vi "IMAQ Multi-camera acquisition of images.vi"() -> ()   [LabVIEW 2018]
uses:
  LabViewDVPCamera/LabViewDVPCamera.lvlib
panel:
  out "Capture frame rate 4":sgl
  out "Total frame rate 4":u32
  out "pFrameCount out 4":T1
  out "Capture frame rate 3":sgl
  out "Total frame rate 3":u32
  out "pFrameCount out 3":T1
  out "Capture frame rate 2":sgl
  out "Total frame rate 2":u32
  out "pFrameCount out 2":T1
  out "Capture frame rate":sgl
  out "Total frame rate":u32
  out "pFrameCount out":T1
  out "frame rate":dbl format="%#.5g"
  out "value 5":u64
  out "Millisecond timing value 7":u32
  out "frame rate":dbl format="%#.5g"
  out "value 4":u64
  out "Millisecond timing value 6":u32
  out "frame rate":dbl format="%#.5g"
  out "数值 3":u64
  out "毫秒计时值 5":u32
  out "frame rate":dbl format="%#.5g"
  out "数值":u64
  out "毫秒计时值 3":u32
  in  "CloseFlg 4":i32
  in  "CameraList 4":u16(ring) caption="CameraList" items=["MGS130M-192.168.0.251"]
  in  "Set 4":bool
  in  "Open 4":bool
  in  "Close 4":bool
  in  "ScanCamera 4":bool
  out "handle 4":u32
  out "Image 4":T2(plugin-control)
  in  "CloseFlg 3":i32
  in  "CameraList 3":u16(ring) caption="CameraList" items=["MGS130M-192.168.0.251"]
  in  "Set 3":bool
  in  "Open 3":bool
  in  "Close 3":bool
  in  "ScanCamera 3":bool
  out "handle 3":u32
  out "Image 3":T2(plugin-control)
  in  "CloseFlg 2":i32
  in  "CameraList 2":u16(ring) caption="CameraList" items=["MGS130M-192.168.0.251"]
  in  "Set 2":bool
  in  "Open 2":bool
  in  "Close 2":bool
  in  "ScanCamera 2":bool
  out "handle 2":u32
  out "Image 2":T2(plugin-control)
  out "Image":T2(plugin-control)
  in  "CloseFlg":i32
  out "handle":u32
  in  "CameraList":u16(ring) items=["MGS130M-192.168.0.251"]
  in  "Set":bool
  in  "Close":bool
  in  "Open":bool
  in  "ScanCamera":bool
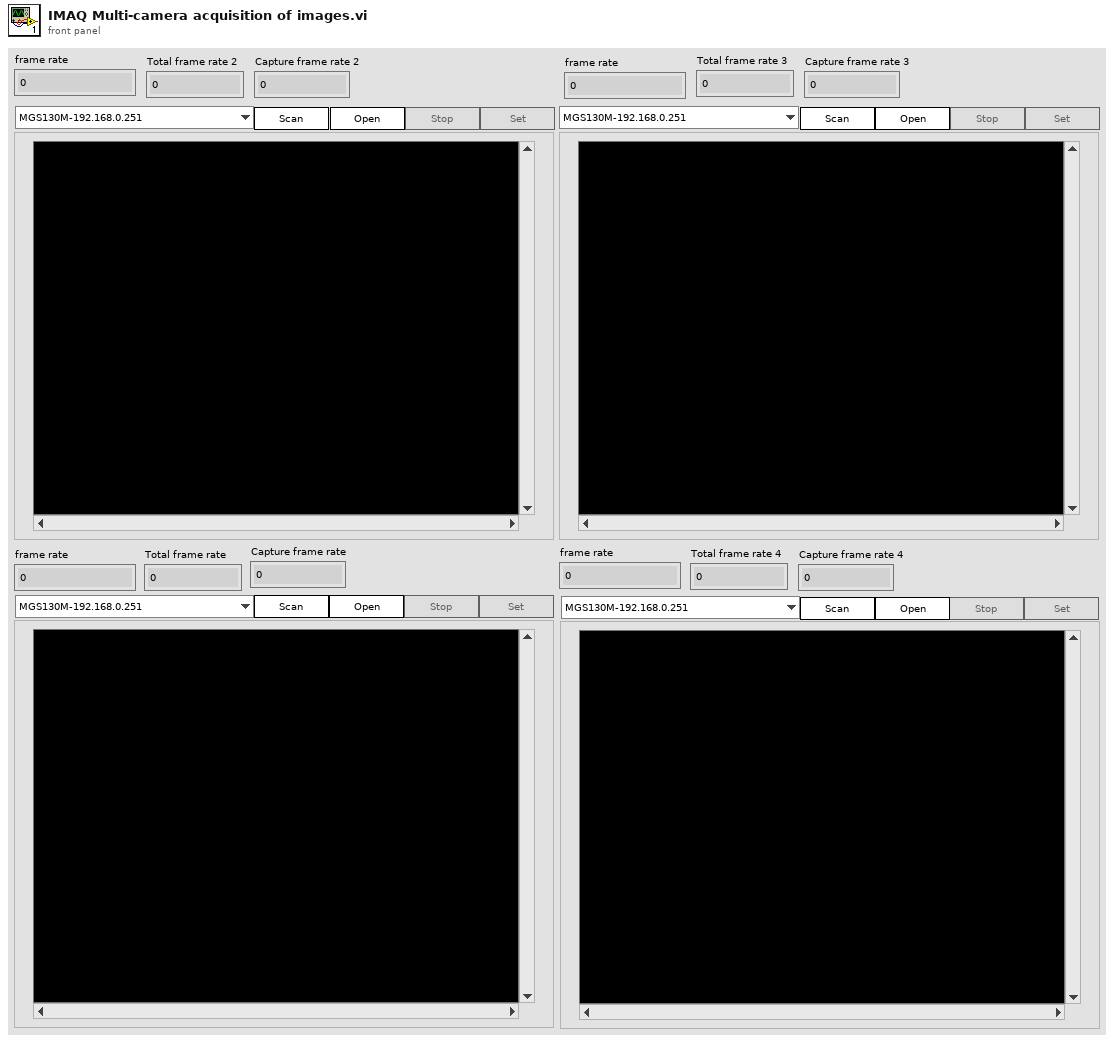
[diagram p1: front panel]
types:
  T1 = cluster{"uFrameCount":u32, "uFrameDrop":u32, "uFrameIgnore":u32, "uFrameError":u32, "uFrameOK":u32, "uFrameOut":u32, "uFrameResend":u32, "uFrameProc":u32, "fFrameRate":sgl, "fProcRate":sgl, "reserved[0]":i32, "reserved[1]":i32, "reserved[2]":i32, "reserved[3]":i32, "reserved[4]":i32, "reserved[5]":i32, "reserved[6]":i32, "reserved[7]":i32, "reserved[8]":i32, "reserved[9]":i32, "reserved[10]":i32, "reserved[11]":i32, "reserved[12]":i32, "reserved[13]":i32, "reserved[14]":i32, "reserved[15]":i32, "reserved[16]":i32, "reserved[17]":i32, "reserved[18]":i32, "reserved[19]":i32, "reserved[20]":i32, "reserved[21]":i32, "reserved[22]":i32, "reserved[23]":i32, "reserved[24]":i32, "reserved[25]":i32, "reserved[26]":i32, "reserved[27]":i32, "reserved[28]":i32, "reserved[29]":i32, "reserved[30]":i32, "reserved[31]":i32}
  T2 = typedef "IMAQ Image.ctl" = refnum<image>
  T3 = enum8{"Enabled", "Disabled", "Disabled and Grayed Out"}
  T4 = typedef "LVStringsAndValuesArrayTypeDef_U16.ctl" = cluster{"String":string, "Value":u16}[]
  T5 = typedef "Image Type" = u32
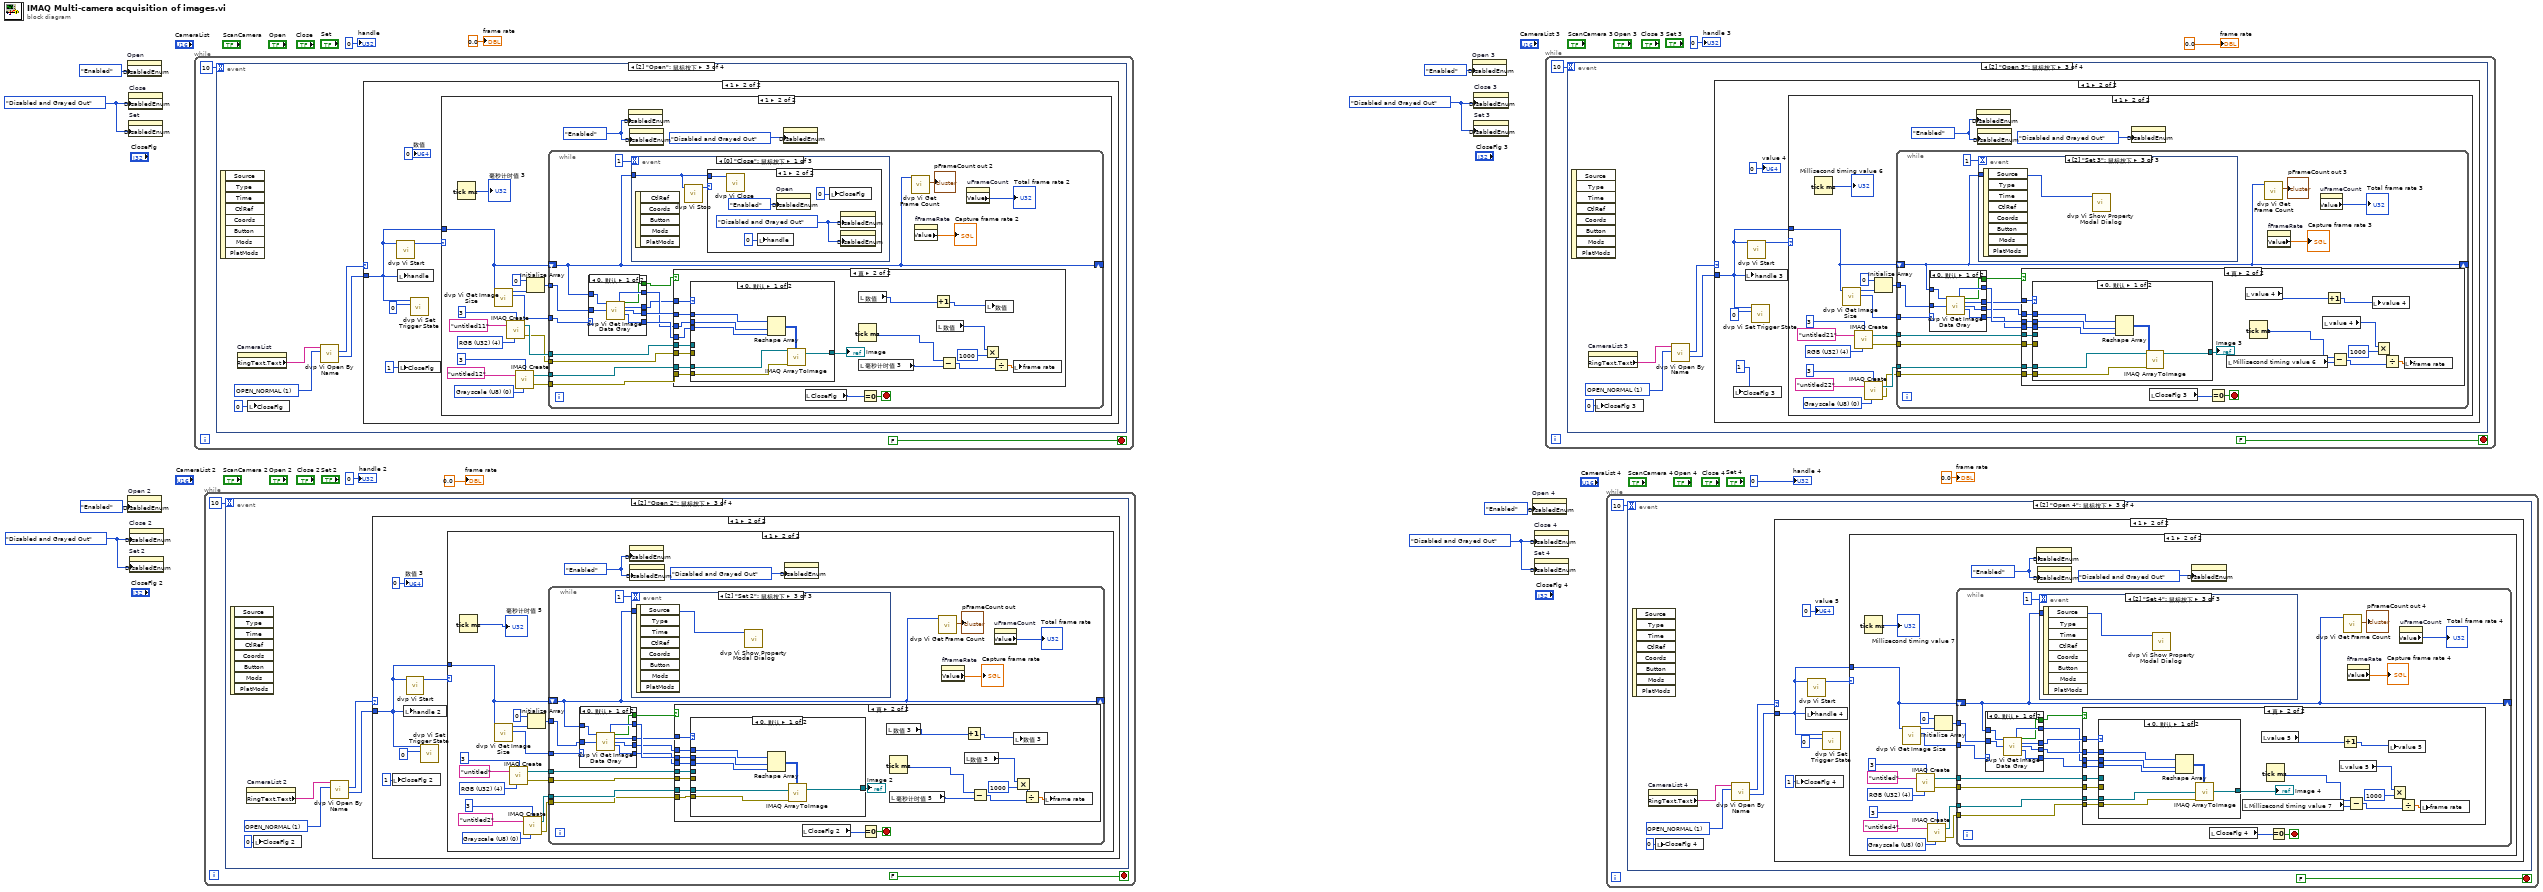
[diagram p0: block diagram]
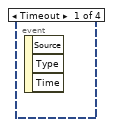
[diagram p2: hidden frame]
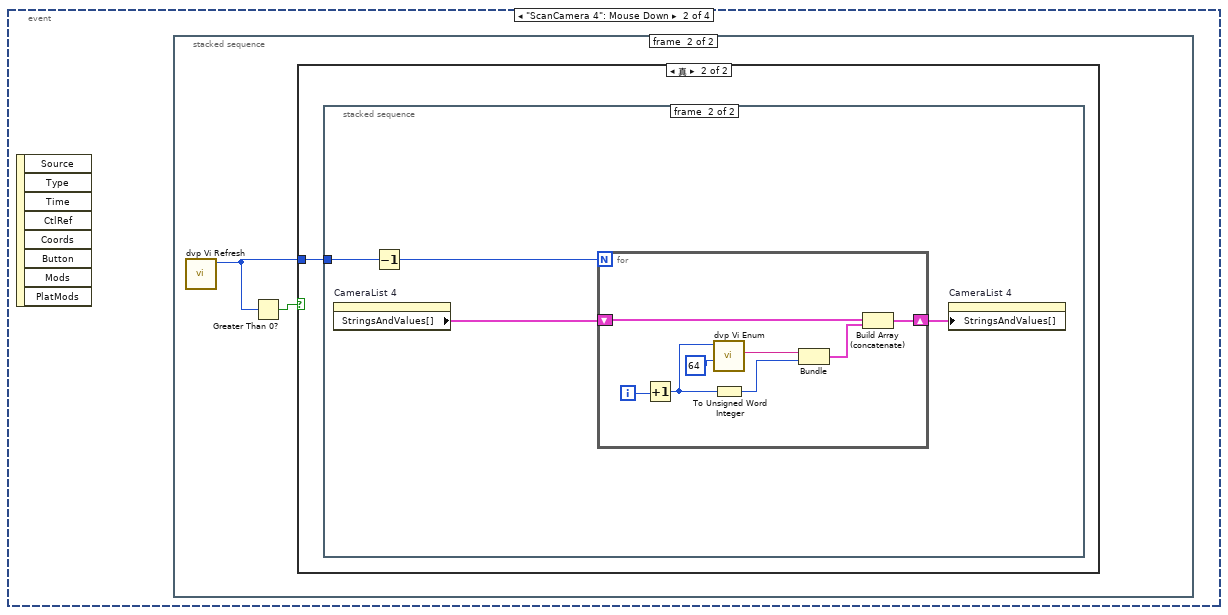
[diagram p3: hidden frame]
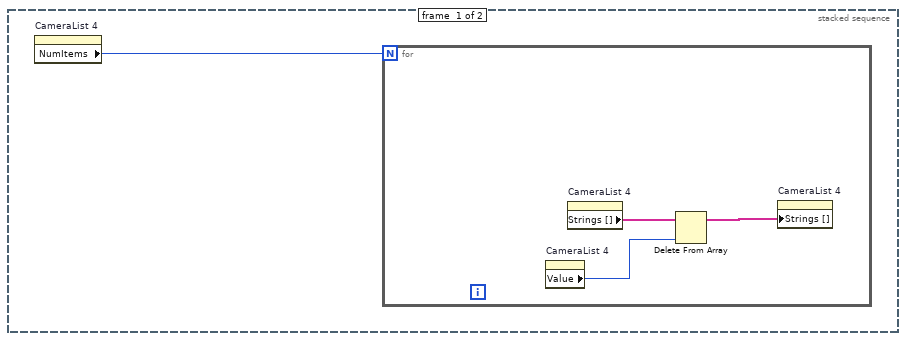
[diagram p4: hidden frame]
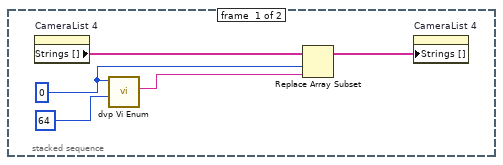
[diagram p6: hidden frame]
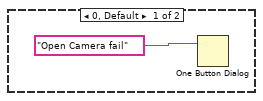
[diagram p7: hidden frame]
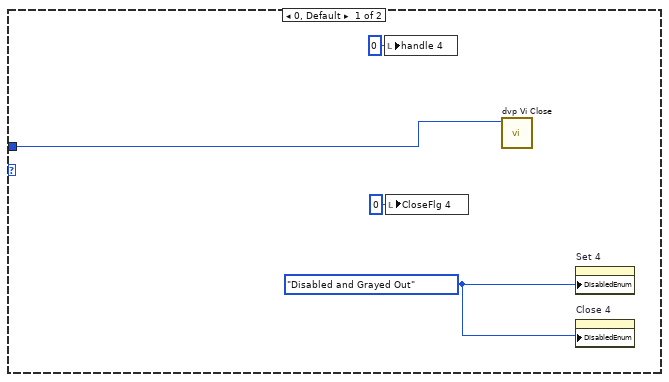
[diagram p8: hidden frame]
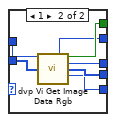
[diagram p9: hidden frame]
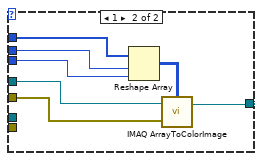
[diagram p11: hidden frame]
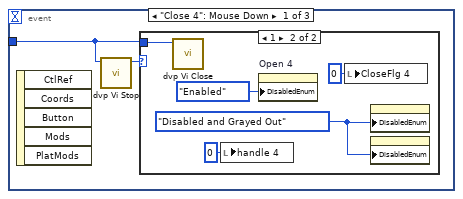
[diagram p12: hidden frame]
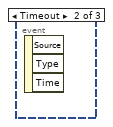
[diagram p14: hidden frame]
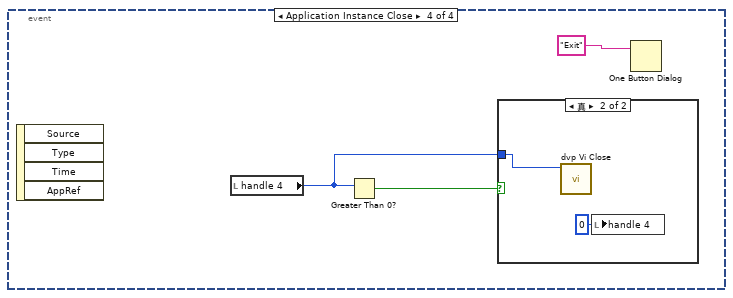
[diagram p15: hidden frame]
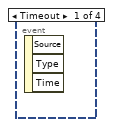
[diagram p17: hidden frame]
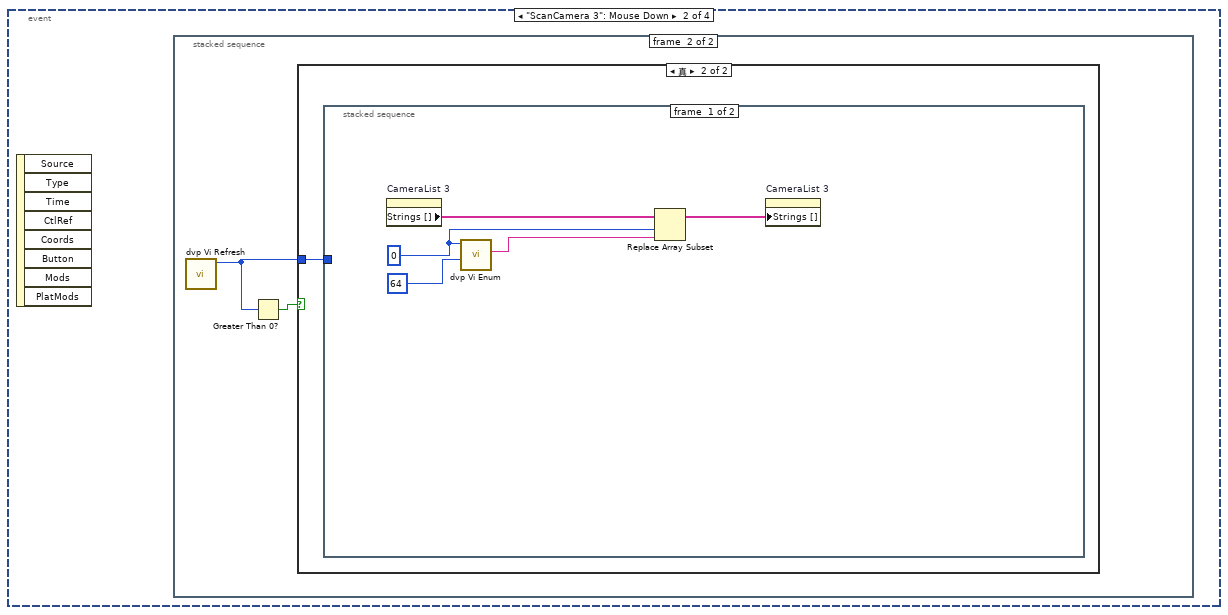
[diagram p18: hidden frame]
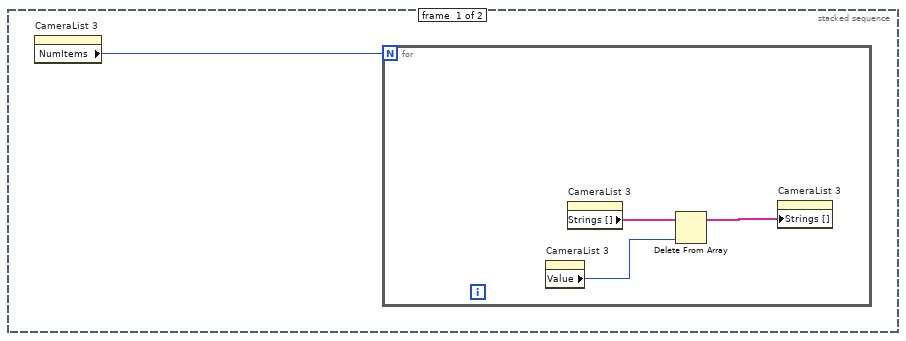
[diagram p19: hidden frame]
diagram:
  w6 = T3."Disabled and Grayed Out" ("禁用")
  w9 = T3."Disabled and Grayed Out" ("禁用")
  w12 = T3."Disabled and Grayed Out" ("禁用")
  w15 = T3."Disabled and Grayed Out" ("禁用")
  n1 = property on="Open" class="Bool"("DisabledEnum"=T3."Enabled" ("禁用")) -> ()  [unwired: 2 in, 2 out]
  n2 = property on="Open 2" class="Bool"("DisabledEnum"=T3."Enabled" ("禁用")) -> ()  [unwired: 2 in, 2 out]
  n3 = property on="Close" class="Bool"("DisabledEnum"=w15) -> ()  [unwired: 2 in, 2 out]
  n4 = property on="Set" class="Bool"("DisabledEnum"=w15) -> ()  [unwired: 2 in, 2 out]
  n5 = property on="Close 2" class="Bool"("DisabledEnum"=w12) -> ()  [unwired: 2 in, 2 out]
  n6 = property on="Set 2" class="Bool"("DisabledEnum"=w12) -> ()  [unwired: 2 in, 2 out]
  n7 = while {
    stop <- FALSE stop-if-true
    n8 = event shown="[2] \"Open\": 鼠标按下" {
      selector: _ -> [_ _ _ _]
      dyn-events: _ -> [_ _ _ _]
      timeout: 10 -> [_ _ _ _]
      event Timeout {
        n9 = event-data() -> ()  [unwired: 1 in, 3 out]
      }
      event "ScanCamera": Mouse Down {
        n10 = event-data() -> ()  [unwired: 1 in, 8 out]
        n11 = stacked-sequence "清除下拉列表的数据" {
          frame #0 {
            n12 = property on="CameraList" class="Ring (严格)"() -> ("NumItems"=w19:u32)  [unwired: 2 in, 2 out]
            n13 = for {
              N: w19 -> [_]
              n14 = property on="CameraList" class="Ring (严格)"() -> ("Value"=w21:u16)  [unwired: 2 in, 2 out]
              n15 = property on="CameraList" class="Ring (严格)"() -> ("Strings []"=w20:string[])  [unwired: 2 in, 2 out]
              n16 = Delete From Array ("删除数组元素")(array=w20, index=w21) -> (array with subset deleted=w22:string[])  [unwired: 1 in, 1 out]
              n17 = property on="CameraList" class="Ring (严格)"("Strings []"=w22) -> ()  [unwired: 2 in, 2 out]
            }
          }
          frame #1 {
            n18 = call "dvp Vi Refresh.vi"() -> ("pCount out"=w24:u32)  [unwired: 10 in, 1 out]
            n19 = Greater Than 0?(x=w24) -> (x > 0?=w23:bool)
            n20 = case shown="真" w23 {
              tunnel: w24 -> [_ w25]
              frame False {
              }
              frame True {
                n21 = stacked-sequence {
                  tunnel: w25 -> [_ w32]
                  frame #0 {
                    w26 = u32 0 ("index")
                    n22 = property on="CameraList" class="Ring (严格)"() -> ("Strings []"=w29:string[])  [unwired: 2 in, 2 out]
                    n23 = call "dvp Vi Enum.vi"("unSize"=u32 64, "index"=w26) -> ("friendlyName out"=w28:string)  [unwired: 8 in, 1 out]
                    n24 = Replace Array Subset ("替换数组子集")(array=w29, new element=w28, index=w26) -> (w30:string[])
                    n25 = property on="CameraList" class="Ring (严格)"("Strings []"=w30) -> ()  [unwired: 2 in, 2 out]
                  }
                  frame #1 {
                    n26 = property on="CameraList" class="Ring (严格)"() -> ("StringsAndValues[]"=w34:T4)  [unwired: 2 in, 2 out]
                    n27 = Decrement(x=w32) -> (x-1=w31:u32)
                    n28 = for {
                      N: w31 -> [_]
                      shift-right: [w41] -> w33
                      shift-left: w34 -> [w39]
                      i -> [w36]
                      n29 = Increment(x=w36) -> (x+1=w35:i32)
                      n30 = call "dvp Vi Enum.vi"("unSize"=u32 64, "index"=w35) -> ("friendlyName out"=w42:string)  [unwired: 8 in, 1 out]
                      n31 = To Unsigned Word Integer(number=w35) -> (unsigned 16bit integer=w38:u16)
                      n32 = Bundle("friendlyName out"=w42, w38) -> (w40:cluster{"friendlyName out":string, u16})  [unwired: 1 in]
                      n33 = Build Array (concatenate) ("创建数组")(w39, w40) -> (w41:T4)
                    }
                    n34 = property on="CameraList" class="Ring (严格)"("StringsAndValues[]"=w33) -> ()  [unwired: 2 in, 2 out]
                  }
                }
              }
            }
          }
        }
      }
      event "Open": Mouse Down {
        w45 = u32 1 items=["OPEN_OFFLINE", "OPEN_NORMAL"] ("type")
        n35 = event-data() -> ()  [unwired: 1 in, 8 out]
        n36 = property on="CameraList" class="Ring (严格)"() -> ("RingText.Text"=w44:string)  [unwired: 2 in, 2 out]
        n37 = local write "CloseFlg"(0 ("CloseFlg")) -> ()
        n38 = call "dvp Vi Open By Name.vi"("type"=w45, "friendlyName"=w44) -> ("pHandle out"=w47:u32, "function return"=w46:u32)  [unwired: 7 in, 1 out]
        n39 = case shown="1" w46 {
          tunnel: w47 -> [_ w50]
          frame 0, Default {
            n40 = One Button Dialog(message="Open Camera fail" ("消息")) -> ()  [unwired: 1 in, 1 out]
          }
          frame 1 {
            n41 = call "dvp Vi Start.vi"("handle"=w50) -> ("function return"=w52:u32)  [unwired: 10 in]
            n42 = local write "handle"(w50) -> ()
            n43 = local write "CloseFlg"(1 ("CloseFlg")) -> ()
            n44 = call "dvp Vi Set Trigger State.vi"("TriggerState"=0, "handle"=w50) -> ()  [unwired: 9 in, 1 out]
            n45 = case shown="1" w52 {
              tunnel: w50 -> [w57 w71]
              frame 0, Default {
                w56 = T3."Disabled and Grayed Out" ("禁用")
                n46 = local write "handle"(u32 0 ("handle")) -> ()
                n47 = local write "CloseFlg"(0 ("CloseFlg")) -> ()
                n48 = call "dvp Vi Close.vi"("handle"=w57) -> ()  [unwired: 10 in, 1 out]
                n49 = property on="Set" class="Bool"("DisabledEnum"=w56) -> ()  [unwired: 2 in, 2 out]
                n50 = property on="Close" class="Bool"("DisabledEnum"=w56) -> ()  [unwired: 2 in, 2 out]
              }
              frame 1 {
                w65 = T5 0 items=["Grayscale (U8)", "Grayscale (I16)", "Grayscale (SGL)", "Complex (CSG)", "RGB (U32)", "HSL (U32)", "RGB (U64)", "Grayscale (U16)"] ("Image Type")
                w69 = T5 4 items=["Grayscale (U8)", "Grayscale (I16)", "Grayscale (SGL)", "Complex (CSG)", "RGB (U32)", "HSL (U32)", "RGB (U64)", "Grayscale (U16)"] ("Image Type")
                w75 = T3."Enabled" ("禁用")
                n51 = Tick Count (ms)() -> (millisecond timer value=→"毫秒计时值 3":u32)
                n52 = call "dvp Vi Get Image Size.vi"("handle"=w71) -> ("pformat out"=w58:i32, "function return"=w70:u32)  [unwired: 9 in]
                n53 = call "IMAQ Create"("Border Size"=3, "Image Name"="untitled11", "Image Type"=w69) -> ("New Image"=w64:T2, "error out"=w61:errorcluster)  [unwired: 2 in]
                n54 = call "IMAQ Create"("Border Size"=3, "Image Name"="untitled12", "Image Type"=w65) -> ("New Image"=w63:T2, "error out"=w62:errorcluster)  [unwired: 2 in]
                n55 = Initialize Array(u8 0 ("元素"), w70) -> (w72:u8[])
                n56 = while {
                  shift-right: [w82] -> _
                  shift-left: w71 -> [w82]
                  tunnel: w72 -> [w83]
                  tunnel: w64 -> [w90]
                  tunnel: w63 -> [w89]
                  tunnel: w62 -> [w88]
                  tunnel: w61 -> [w87]
                  tunnel: w58 -> [w81]
                  stop <- w92 stop-if-true
                  n57 = case shown="0, 默认" w81 {
                    tunnel: w83 -> [w100 w107]
                    tunnel: w82 -> [w99 w106]
                    tunnel: [w95 w105] -> w79
                    tunnel: [w97 w104] -> w80
                    tunnel: [w96 w103] -> w76
                    tunnel: [w98 w102] -> w77
                    tunnel: [w94 w101] -> w78
                    frame 0, Default {
                      n58 = call "dvp Vi Get Image Data Gray.vi"("handle"=w99, "pbuffer"=w100) -> ("piHeight out"=w98:i32, "function return"=w95:bool, "pformat out"=w96:i32, "pbuffer out"=w97:u8[], "piWidth out"=w94:i32)  [unwired: 9 in]
                    }
                    frame 1 {
                      n59 = call "dvp Vi Get Image Data Rgb.vi"("handle"=w106, "pbuffer"=w107) -> ("piHeight out"=w102:i32, "function return"=w105:bool, "pformat out"=w103:i32, "pbuffer out"=w104:u32[], "piWidth out"=w101:i32)  [unwired: 9 in]
                    }
                  }
                  n60 = event shown="[0] \"Close\": 鼠标按下" {
                    selector: _ -> [_ _ _]
                    dyn-events: _ -> [_ _ _]
                    timeout: 1 -> [_ _ _]
                    tunnel: w82 -> [w140 _ w147]
                    event "Close": Mouse Down {
                      n61 = event-data() -> ()  [unwired: 1 in, 5 out]
                      n62 = call "dvp Vi Stop.vi"("handle"=w140) -> ("function return"=w141:u32)  [unwired: 10 in]
                      n63 = case shown="1" w141 {
                        tunnel: w140 -> [_ w144]
                        frame 0, Default {
                        }
                        frame 1 {
                          w143 = T3."Disabled and Grayed Out" ("禁用")
                          n64 = call "dvp Vi Close.vi"("handle"=w144) -> ()  [unwired: 10 in, 1 out]
                          n65 = local write "handle"(u32 0 ("handle")) -> ()
                          n66 = property on="Open" class="Bool"("DisabledEnum"=T3."Enabled" ("禁用")) -> ()  [unwired: 2 in, 2 out]
                          n67 = local write "CloseFlg"(0 ("CloseFlg")) -> ()
                          n68 = property on="Close" class="Bool"("DisabledEnum"=w143) -> ()  [unwired: 2 in, 2 out]
                          n69 = property on="Set" class="Bool"("DisabledEnum"=w143) -> ()  [unwired: 2 in, 2 out]
                        }
                      }
                    }
                    event Timeout {
                      n70 = event-data() -> ()  [unwired: 1 in, 3 out]
                    }
                    event "Set": Mouse Down {
                      n71 = event-data() -> ()  [unwired: 1 in, 8 out]
                      n72 = call "dvp Vi Show Property Modal Dialog.vi"("handle"=w147) -> ()  [unwired: 10 in, 1 out]
                    }
                  }
                  n73 = case shown="真" w79 {
                    tunnel: w78 -> [_ w125]
                    tunnel: w77 -> [_ w124]
                    tunnel: w80 -> [_ w123]
                    tunnel: w76 -> [_ w122]
                    tunnel: w90 -> [_ w118]
                    tunnel: w89 -> [_ w121]
                    tunnel: w88 -> [_ w120]
                    tunnel: w87 -> [_ w119]
                    frame False {
                    }
                    frame True {
                      n74 = case shown="0, 默认" w122 {
                        tunnel: w124 -> [w132 w138]
                        tunnel: w125 -> [w131 w139]
                        tunnel: [w130 w136] -> w117
                        tunnel: w123 -> [w126 w135]
                        tunnel: w121 -> [w127 _]
                        tunnel: w120 -> [w128 _]
                        tunnel: w119 -> [_ w133]
                        tunnel: w118 -> [_ w134]
                        frame 0, Default {
                          n75 = Reshape Array ("重排数组维数")(w126, w132, w131) -> (w129:u32[][])
                          n76 = call "IMAQ ArrayToImage"("error in (no error)"=w128, "Image Pixels (U8)"=w129, "Image"=w127) -> ("Image Out"=w130:T2)  [unwired: 7 in, 1 out]
                        }
                        frame 1 {
                          n77 = Reshape Array ("重排数组维数")(w135, w138, w139) -> (w137:u32[][])
                          n78 = call "IMAQ ArrayToColorImage"("Image Pixels (U32)"=w137, "Image"=w134, "error in (no error)"=w133) -> ("Image Out"=w136:T2)  [unwired: 2 in, 1 out]
                        }
                      }
                      "Image" <- w117
                      n79 = local read "数值"() -> (w111:u64)
                      n80 = Tick Count (ms)() -> (millisecond timer value=w113:u32)
                      n81 = local read "毫秒计时值 3"() -> (w114:u32)
                      n82 = Increment(x=w111) -> (x+1=w112:u64)
                      n83 = local read "数值"() -> (w115:u64)
                      n84 = Subtract(x=w113, y=w114) -> (x-y=w108:u32)
                      n85 = Multiply(x=w115, y=u64 1000) -> (x*y=w110:u64)
                      n86 = local write "数值"(w112) -> ()
                      n87 = Divide(x=w110, y=w108) -> (x/y=w116:dbl)
                      n88 = local write "frame rate"(w116) -> ()
                    }
                  }
                  n89 = local read "CloseFlg"() -> (w91:i32)
                  n90 = Equal To 0?(x=w91) -> (x = 0?=w92:bool)
                  n91 = call "dvp Vi Get Frame Count.vi"("handle"=w82) -> ("pFrameCount out"=→"pFrameCount out 2":T1)  [unwired: 9 in, 1 out]
                  n92 = property on="fFrameRate" class="DigNum (严格)"() -> ("Value"=→"Capture frame rate 2":sgl)  [unwired: 2 in, 2 out]
                  n93 = property on="uFrameCount" class="DigNum (严格)"() -> ("Value"=→"Total frame rate 2":u32)  [unwired: 2 in, 2 out]
                }
                n94 = property on="Set" class="Bool"("DisabledEnum"=w75) -> ()  [unwired: 2 in, 2 out]
                n95 = property on="Close" class="Bool"("DisabledEnum"=w75) -> ()  [unwired: 2 in, 2 out]
                n96 = property on="Open" class="Bool"("DisabledEnum"=T3."Disabled and Grayed Out" ("禁用")) -> ()  [unwired: 2 in, 2 out]
              }
            }
            "数值" <- u64 0 ("数值")
          }
        }
      }
      event Application Instance Close {
        n97 = event-data() -> ()  [unwired: 1 in, 4 out]
        n98 = local read "handle"() -> (w148:u32)
        n99 = Greater Than 0?(x=w148) -> (x > 0?=w149:bool)
        n100 = case shown="真" w149 {
          tunnel: w148 -> [_ w152]
          frame False {
          }
          frame True {
            n101 = call "dvp Vi Close.vi"("handle"=w152) -> ()  [unwired: 10 in, 1 out]
            n102 = local write "handle"(u32 0 ("handle")) -> ()
          }
        }
        n103 = One Button Dialog(message="Exit" ("消息")) -> ()  [unwired: 1 in, 1 out]
      }
    }
  }
  n104 = while {
    stop <- FALSE stop-if-true
    n105 = event shown="[2] \"Open 2\": 鼠标按下" {
      selector: _ -> [_ _ _ _]
      dyn-events: _ -> [_ _ _ _]
      timeout: 10 -> [_ _ _ _]
      event Timeout {
        n106 = event-data() -> ()  [unwired: 1 in, 3 out]
      }
      event "ScanCamera 2": Mouse Down {
        n107 = event-data() -> ()  [unwired: 1 in, 8 out]
        n108 = stacked-sequence "清除下拉列表的数据" {
          frame #0 {
            n109 = property on="CameraList 2" class="Ring (严格)"() -> ("NumItems"=w155:u32)  [unwired: 2 in, 2 out]
            n110 = for {
              N: w155 -> [_]
              n111 = property on="CameraList 2" class="Ring (严格)"() -> ("Value"=w157:u16)  [unwired: 2 in, 2 out]
              n112 = property on="CameraList 2" class="Ring (严格)"() -> ("Strings []"=w156:string[])  [unwired: 2 in, 2 out]
              n113 = Delete From Array ("删除数组元素")(array=w156, index=w157) -> (array with subset deleted=w158:string[])  [unwired: 1 in, 1 out]
              n114 = property on="CameraList 2" class="Ring (严格)"("Strings []"=w158) -> ()  [unwired: 2 in, 2 out]
            }
          }
          frame #1 {
            n115 = call "dvp Vi Refresh.vi"() -> ("pCount out"=w160:u32)  [unwired: 10 in, 1 out]
            n116 = Greater Than 0?(x=w160) -> (x > 0?=w159:bool)
            n117 = case shown="真" w159 {
              tunnel: w160 -> [_ w161]
              frame False {
              }
              frame True {
                n118 = stacked-sequence {
                  tunnel: w161 -> [_ w168]
                  frame #0 {
                    w162 = u32 0 ("index")
                    n119 = property on="CameraList 2" class="Ring (严格)"() -> ("Strings []"=w165:string[])  [unwired: 2 in, 2 out]
                    n120 = call "dvp Vi Enum.vi"("unSize"=u32 64, "index"=w162) -> ("friendlyName out"=w164:string)  [unwired: 8 in, 1 out]
                    n121 = Replace Array Subset ("替换数组子集")(array=w165, new element=w164, index=w162) -> (w166:string[])
                    n122 = property on="CameraList 2" class="Ring (严格)"("Strings []"=w166) -> ()  [unwired: 2 in, 2 out]
                  }
                  frame #1 {
                    n123 = property on="CameraList 2" class="Ring (严格)"() -> ("StringsAndValues[]"=w170:T4)  [unwired: 2 in, 2 out]
                    n124 = Decrement(x=w168) -> (x-1=w167:u32)
                    n125 = for {
                      N: w167 -> [_]
                      shift-right: [w177] -> w169
                      shift-left: w170 -> [w175]
                      i -> [w172]
                      n126 = Increment(x=w172) -> (x+1=w171:i32)
                      n127 = call "dvp Vi Enum.vi"("unSize"=u32 64, "index"=w171) -> ("friendlyName out"=w178:string)  [unwired: 8 in, 1 out]
                      n128 = To Unsigned Word Integer(number=w171) -> (unsigned 16bit integer=w174:u16)
                      n129 = Bundle("friendlyName out"=w178, w174) -> (w176:cluster{"friendlyName out":string, u16})  [unwired: 1 in]
                      n130 = Build Array (concatenate) ("创建数组")(w175, w176) -> (w177:T4)
                    }
                    n131 = property on="CameraList 2" class="Ring (严格)"("StringsAndValues[]"=w169) -> ()  [unwired: 2 in, 2 out]
                  }
                }
              }
            }
          }
        }
      }
      event "Open 2": Mouse Down {
        w181 = u32 1 items=["OPEN_OFFLINE", "OPEN_NORMAL"] ("type")
        n132 = event-data() -> ()  [unwired: 1 in, 8 out]
        n133 = property on="CameraList 2" class="Ring (严格)"() -> ("RingText.Text"=w180:string)  [unwired: 2 in, 2 out]
        n134 = local write "CloseFlg 2"(0 ("CloseFlg")) -> ()
        n135 = call "dvp Vi Open By Name.vi"("type"=w181, "friendlyName"=w180) -> ("pHandle out"=w183:u32, "function return"=w182:u32)  [unwired: 7 in, 1 out]
        n136 = case shown="1" w182 {
          tunnel: w183 -> [_ w186]
          frame 0, Default {
            n137 = One Button Dialog(message="Open Camera fail" ("消息")) -> ()  [unwired: 1 in, 1 out]
          }
          frame 1 {
            n138 = local write "CloseFlg 2"(1 ("CloseFlg")) -> ()
            n139 = local write "handle 2"(w186) -> ()
            n140 = call "dvp Vi Start.vi"("handle"=w186) -> ("function return"=w188:u32)  [unwired: 10 in]
            n141 = call "dvp Vi Set Trigger State.vi"("TriggerState"=0, "handle"=w186) -> ()  [unwired: 9 in, 1 out]
            n142 = case shown="1" w188 {
              tunnel: w186 -> [w193 w207]
              frame 0, Default {
                w192 = T3."Disabled and Grayed Out" ("禁用")
                n143 = local write "handle 2"(u32 0 ("handle")) -> ()
                n144 = local write "CloseFlg 2"(0 ("CloseFlg")) -> ()
                n145 = call "dvp Vi Close.vi"("handle"=w193) -> ()  [unwired: 10 in, 1 out]
                n146 = property on="Set 2" class="Bool"("DisabledEnum"=w192) -> ()  [unwired: 2 in, 2 out]
                n147 = property on="Close 2" class="Bool"("DisabledEnum"=w192) -> ()  [unwired: 2 in, 2 out]
              }
              frame 1 {
                w202 = T5 4 items=["Grayscale (U8)", "Grayscale (I16)", "Grayscale (SGL)", "Complex (CSG)", "RGB (U32)", "HSL (U32)", "RGB (U64)", "Grayscale (U16)"] ("Image Type")
                w205 = T5 0 items=["Grayscale (U8)", "Grayscale (I16)", "Grayscale (SGL)", "Complex (CSG)", "RGB (U32)", "HSL (U32)", "RGB (U64)", "Grayscale (U16)"] ("Image Type")
                w211 = T3."Enabled" ("禁用")
                n148 = Tick Count (ms)() -> (millisecond timer value=→"毫秒计时值 5":u32)
                n149 = call "dvp Vi Get Image Size.vi"("handle"=w207) -> ("pformat out"=w194:i32, "function return"=w206:u32)  [unwired: 9 in]
                n150 = call "IMAQ Create"("Border Size"=3, "Image Name"="untitled", "Image Type"=w202) -> ("New Image"=w199:T2, "error out"=w198:errorcluster)  [unwired: 2 in]
                n151 = call "IMAQ Create"("Border Size"=3, "Image Name"="untitled2", "Image Type"=w205) -> ("New Image"=w197:T2, "error out"=w196:errorcluster)  [unwired: 2 in]
                n152 = Initialize Array(u8 0 ("元素"), w206) -> (w208:u8[])
                n153 = while {
                  shift-right: [w218] -> _
                  shift-left: w207 -> [w218]
                  tunnel: w208 -> [w212]
                  tunnel: w199 -> [w226]
                  tunnel: w198 -> [w225]
                  tunnel: w197 -> [w224]
                  tunnel: w196 -> [w223]
                  tunnel: w194 -> [w219]
                  stop <- w228 stop-if-true
                  n154 = case shown="0, 默认" w219 {
                    tunnel: w212 -> [w236 w243]
                    tunnel: w218 -> [w235 w242]
                    tunnel: [w231 w241] -> w217
                    tunnel: [w233 w240] -> w213
                    tunnel: [w232 w239] -> w214
                    tunnel: [w234 w238] -> w216
                    tunnel: [w230 w237] -> w215
                    frame 0, Default {
                      n155 = call "dvp Vi Get Image Data Gray.vi"("handle"=w235, "pbuffer"=w236) -> ("piHeight out"=w234:i32, "function return"=w231:bool, "pformat out"=w232:i32, "pbuffer out"=w233:u8[], "piWidth out"=w230:i32)  [unwired: 9 in]
                    }
                    frame 1 {
                      n156 = call "dvp Vi Get Image Data Rgb.vi"("handle"=w242, "pbuffer"=w243) -> ("piHeight out"=w238:i32, "function return"=w241:bool, "pformat out"=w239:i32, "pbuffer out"=w240:u32[], "piWidth out"=w237:i32)  [unwired: 9 in]
                    }
                  }
                  n157 = event shown="[2] \"Set 2\": 鼠标按下" {
                    selector: _ -> [_ _ _]
                    dyn-events: _ -> [_ _ _]
                    timeout: 1 -> [_ _ _]
                    tunnel: w218 -> [w276 _ w283]
                    event "Close 2": Mouse Down {
                      n158 = event-data() -> ()  [unwired: 1 in, 5 out]
                      n159 = call "dvp Vi Stop.vi"("handle"=w276) -> ("function return"=w277:u32)  [unwired: 10 in]
                      n160 = case shown="1" w277 {
                        tunnel: w276 -> [_ w280]
                        frame 0, Default {
                        }
                        frame 1 {
                          w279 = T3."Disabled and Grayed Out" ("禁用")
                          n161 = call "dvp Vi Close.vi"("handle"=w280) -> ()  [unwired: 10 in, 1 out]
                          n162 = local write "handle 2"(u32 0 ("handle")) -> ()
                          n163 = property on="Open 2" class="Bool"("DisabledEnum"=T3."Enabled" ("禁用")) -> ()  [unwired: 2 in, 2 out]
                          n164 = local write "CloseFlg 2"(0 ("CloseFlg")) -> ()
                          n165 = property on="Close 2" class="Bool"("DisabledEnum"=w279) -> ()  [unwired: 2 in, 2 out]
                          n166 = property on="Set 2" class="Bool"("DisabledEnum"=w279) -> ()  [unwired: 2 in, 2 out]
                        }
                      }
                    }
                    event Timeout {
                      n167 = event-data() -> ()  [unwired: 1 in, 3 out]
                    }
                    event "Set 2": Mouse Down {
                      n168 = event-data() -> ()  [unwired: 1 in, 8 out]
                      n169 = call "dvp Vi Show Property Modal Dialog.vi"("handle"=w283) -> ()  [unwired: 10 in, 1 out]
                    }
                  }
                  n170 = case shown="真" w217 {
                    tunnel: w215 -> [_ w261]
                    tunnel: w216 -> [_ w260]
                    tunnel: w213 -> [_ w258]
                    tunnel: w214 -> [_ w257]
                    tunnel: w226 -> [_ w256]
                    tunnel: w225 -> [_ w255]
                    tunnel: w224 -> [_ w254]
                    tunnel: w223 -> [_ w253]
                    frame False {
                    }
                    frame True {
                      n171 = case shown="0, 默认" w257 {
                        tunnel: w260 -> [w268 w274]
                        tunnel: w261 -> [w267 w275]
                        tunnel: [w266 w272] -> w259
                        tunnel: w258 -> [w262 w271]
                        tunnel: w256 -> [_ w270]
                        tunnel: w255 -> [_ w269]
                        tunnel: w254 -> [w263 _]
                        tunnel: w253 -> [w264 _]
                        frame 0, Default {
                          n172 = Reshape Array ("重排数组维数")(w262, w268, w267) -> (w265:u32[][])
                          n173 = call "IMAQ ArrayToImage"("error in (no error)"=w264, "Image Pixels (U8)"=w265, "Image"=w263) -> ("Image Out"=w266:T2)  [unwired: 7 in, 1 out]
                        }
                        frame 1 {
                          n174 = Reshape Array ("重排数组维数")(w271, w274, w275) -> (w273:u32[][])
                          n175 = call "IMAQ ArrayToColorImage"("Image Pixels (U32)"=w273, "Image"=w270, "error in (no error)"=w269) -> ("Image Out"=w272:T2)  [unwired: 2 in, 1 out]
                        }
                      }
                      "Image 2" <- w259
                      n176 = local read "数值 3"() -> (w249:u64)
                      n177 = Tick Count (ms)() -> (millisecond timer value=w247:u32)
                      n178 = local read "毫秒计时值 5"() -> (w246:u32)
                      n179 = local read "数值 3"() -> (w245:u64)
                      n180 = Increment(x=w249) -> (x+1=w248:u64)
                      n181 = Subtract(x=w247, y=w246) -> (x-y=w252:u32)
                      n182 = local write "数值 3"(w248) -> ()
                      n183 = Multiply(x=w245, y=u64 1000) -> (x*y=w250:u64)
                      n184 = Divide(x=w250, y=w252) -> (x/y=w244:dbl)
                      n185 = local write "frame rate"(w244) -> ()
                    }
                  }
                  n186 = local read "CloseFlg 2"() -> (w227:i32)
                  n187 = Equal To 0?(x=w227) -> (x = 0?=w228:bool)
                  n188 = call "dvp Vi Get Frame Count.vi"("handle"=w218) -> ("pFrameCount out"=→"pFrameCount out":T1)  [unwired: 9 in, 1 out]
                  n189 = property on="fFrameRate" class="DigNum (严格)"() -> ("Value"=→"Capture frame rate":sgl)  [unwired: 2 in, 2 out]
                  n190 = property on="uFrameCount" class="DigNum (严格)"() -> ("Value"=→"Total frame rate":u32)  [unwired: 2 in, 2 out]
                }
                n191 = property on="Set 2" class="Bool"("DisabledEnum"=w211) -> ()  [unwired: 2 in, 2 out]
                n192 = property on="Close 2" class="Bool"("DisabledEnum"=w211) -> ()  [unwired: 2 in, 2 out]
                n193 = property on="Open 2" class="Bool"("DisabledEnum"=T3."Disabled and Grayed Out" ("禁用")) -> ()  [unwired: 2 in, 2 out]
              }
            }
            "数值 3" <- u64 0 ("数值 3")
          }
        }
      }
      event Application Instance Close {
        n194 = event-data() -> ()  [unwired: 1 in, 4 out]
        n195 = local read "handle 2"() -> (w284:u32)
        n196 = Greater Than 0?(x=w284) -> (x > 0?=w285:bool)
        n197 = case shown="真" w285 {
          tunnel: w284 -> [_ w288]
          frame False {
          }
          frame True {
            n198 = call "dvp Vi Close.vi"("handle"=w288) -> ()  [unwired: 10 in, 1 out]
            n199 = local write "handle 2"(u32 0 ("handle")) -> ()
          }
        }
        n200 = One Button Dialog(message="Exit" ("消息")) -> ()  [unwired: 1 in, 1 out]
      }
    }
  }
  n201 = property on="Open 3" class="Bool"("DisabledEnum"=T3."Enabled" ("禁用")) -> ()  [unwired: 2 in, 2 out]
  n202 = property on="Close 3" class="Bool"("DisabledEnum"=w9) -> ()  [unwired: 2 in, 2 out]
  n203 = property on="Set 3" class="Bool"("DisabledEnum"=w9) -> ()  [unwired: 2 in, 2 out]
  n204 = property on="Open 4" class="Bool"("DisabledEnum"=T3."Enabled" ("禁用")) -> ()  [unwired: 2 in, 2 out]
  n205 = property on="Close 4" class="Bool"("DisabledEnum"=w6) -> ()  [unwired: 2 in, 2 out]
  n206 = property on="Set 4" class="Bool"("DisabledEnum"=w6) -> ()  [unwired: 2 in, 2 out]
  n207 = while {
    stop <- FALSE stop-if-true
    n208 = event shown="[2] \"Open 3\": 鼠标按下" {
      selector: _ -> [_ _ _ _]
      dyn-events: _ -> [_ _ _ _]
      timeout: 10 -> [_ _ _ _]
      event Timeout {
        n209 = event-data() -> ()  [unwired: 1 in, 3 out]
      }
      event "ScanCamera 3": Mouse Down {
        n210 = event-data() -> ()  [unwired: 1 in, 8 out]
        n211 = stacked-sequence "清除下拉列表的数据" {
          frame #0 {
            n212 = property on="CameraList 3" class="Ring (严格)"() -> ("NumItems"=w291:u32)  [unwired: 2 in, 2 out]
            n213 = for {
              N: w291 -> [_]
              n214 = property on="CameraList 3" class="Ring (严格)"() -> ("Value"=w293:u16)  [unwired: 2 in, 2 out]
              n215 = property on="CameraList 3" class="Ring (严格)"() -> ("Strings []"=w292:string[])  [unwired: 2 in, 2 out]
              n216 = Delete From Array ("删除数组元素")(array=w292, index=w293) -> (array with subset deleted=w294:string[])  [unwired: 1 in, 1 out]
              n217 = property on="CameraList 3" class="Ring (严格)"("Strings []"=w294) -> ()  [unwired: 2 in, 2 out]
            }
          }
          frame #1 {
            n218 = call "dvp Vi Refresh.vi"() -> ("pCount out"=w296:u32)  [unwired: 10 in, 1 out]
            n219 = Greater Than 0?(x=w296) -> (x > 0?=w295:bool)
            n220 = case shown="真" w295 {
              tunnel: w296 -> [_ w297]
              frame False {
              }
              frame True {
                n221 = stacked-sequence {
                  tunnel: w297 -> [_ w304]
                  frame #0 {
                    w298 = u32 0 ("index")
                    n222 = property on="CameraList 3" class="Ring (严格)"() -> ("Strings []"=w301:string[])  [unwired: 2 in, 2 out]
                    n223 = call "dvp Vi Enum.vi"("unSize"=u32 64, "index"=w298) -> ("friendlyName out"=w300:string)  [unwired: 8 in, 1 out]
                    n224 = Replace Array Subset ("替换数组子集")(array=w301, new element=w300, index=w298) -> (w302:string[])
                    n225 = property on="CameraList 3" class="Ring (严格)"("Strings []"=w302) -> ()  [unwired: 2 in, 2 out]
                  }
                  frame #1 {
                    n226 = property on="CameraList 3" class="Ring (严格)"() -> ("StringsAndValues[]"=w306:T4)  [unwired: 2 in, 2 out]
                    n227 = Decrement(x=w304) -> (x-1=w303:u32)
                    n228 = for {
                      N: w303 -> [_]
                      shift-right: [w313] -> w305
                      shift-left: w306 -> [w311]
                      i -> [w308]
                      n229 = Increment(x=w308) -> (x+1=w307:i32)
                      n230 = call "dvp Vi Enum.vi"("unSize"=u32 64, "index"=w307) -> ("friendlyName out"=w314:string)  [unwired: 8 in, 1 out]
                      n231 = To Unsigned Word Integer(number=w307) -> (unsigned 16bit integer=w310:u16)
                      n232 = Bundle("friendlyName out"=w314, w310) -> (w312:cluster{"friendlyName out":string, u16})  [unwired: 1 in]
                      n233 = Build Array (concatenate) ("创建数组")(w311, w312) -> (w313:T4)
                    }
                    n234 = property on="CameraList 3" class="Ring (严格)"("StringsAndValues[]"=w305) -> ()  [unwired: 2 in, 2 out]
                  }
                }
              }
            }
          }
        }
      }
      event "Open 3": Mouse Down {
        w317 = u32 1 items=["OPEN_OFFLINE", "OPEN_NORMAL"] ("type")
        n235 = event-data() -> ()  [unwired: 1 in, 8 out]
        n236 = property on="CameraList 3" class="Ring (严格)"() -> ("RingText.Text"=w316:string)  [unwired: 2 in, 2 out]
        n237 = local write "CloseFlg 3"(0 ("CloseFlg")) -> ()
        n238 = call "dvp Vi Open By Name.vi"("type"=w317, "friendlyName"=w316) -> ("pHandle out"=w319:u32, "function return"=w318:u32)  [unwired: 7 in, 1 out]
        n239 = case shown="1" w318 {
          tunnel: w319 -> [_ w322]
          frame 0, Default {
            n240 = One Button Dialog(message="Open Camera fail" ("消息")) -> ()  [unwired: 1 in, 1 out]
          }
          frame 1 {
            n241 = local write "CloseFlg 3"(1 ("CloseFlg")) -> ()
            n242 = local write "handle 3"(w322) -> ()
            n243 = call "dvp Vi Start.vi"("handle"=w322) -> ("function return"=w324:u32)  [unwired: 10 in]
            n244 = call "dvp Vi Set Trigger State.vi"("TriggerState"=0, "handle"=w322) -> ()  [unwired: 9 in, 1 out]
            n245 = case shown="1" w324 {
              tunnel: w322 -> [w329 w343]
              frame 0, Default {
                w328 = T3."Disabled and Grayed Out" ("禁用")
                n246 = local write "handle 3"(u32 0 ("handle")) -> ()
                n247 = local write "CloseFlg 3"(0 ("CloseFlg")) -> ()
                n248 = call "dvp Vi Close.vi"("handle"=w329) -> ()  [unwired: 10 in, 1 out]
                n249 = property on="Set 3" class="Bool"("DisabledEnum"=w328) -> ()  [unwired: 2 in, 2 out]
                n250 = property on="Close 3" class="Bool"("DisabledEnum"=w328) -> ()  [unwired: 2 in, 2 out]
              }
              frame 1 {
                w339 = T5 0 items=["Grayscale (U8)", "Grayscale (I16)", "Grayscale (SGL)", "Complex (CSG)", "RGB (U32)", "HSL (U32)", "RGB (U64)", "Grayscale (U16)"] ("Image Type")
                w341 = T5 4 items=["Grayscale (U8)", "Grayscale (I16)", "Grayscale (SGL)", "Complex (CSG)", "RGB (U32)", "HSL (U32)", "RGB (U64)", "Grayscale (U16)"] ("Image Type")
                w347 = T3."Enabled" ("禁用")
                n251 = Tick Count (ms)() -> (millisecond timer value=→"Millisecond timing value 6":u32)
                n252 = call "dvp Vi Get Image Size.vi"("handle"=w343) -> ("pformat out"=w330:i32, "function return"=w342:u32)  [unwired: 9 in]
                n253 = call "IMAQ Create"("Border Size"=3, "Image Name"="untitled21", "Image Type"=w341) -> ("New Image"=w333:T2, "error out"=w332:errorcluster)  [unwired: 2 in]
                n254 = call "IMAQ Create"("Border Size"=3, "Image Name"="untitled22", "Image Type"=w339) -> ("New Image"=w335:T2, "error out"=w334:errorcluster)  [unwired: 2 in]
                n255 = Initialize Array(u8 0 ("元素"), w342) -> (w344:u8[])
                n256 = while {
                  shift-right: [w355] -> _
                  shift-left: w343 -> [w355]
                  tunnel: w344 -> [w354]
                  tunnel: w335 -> [w362]
                  tunnel: w334 -> [w361]
                  tunnel: w333 -> [w360]
                  tunnel: w332 -> [w359]
                  tunnel: w330 -> [w353]
                  stop <- w364 stop-if-true
                  n257 = case shown="0, 默认" w353 {
                    tunnel: w354 -> [w372 w379]
                    tunnel: w355 -> [w371 w378]
                    tunnel: [w367 w377] -> w352
                    tunnel: [w369 w376] -> w350
                    tunnel: [w368 w375] -> w349
                    tunnel: [w370 w374] -> w351
                    tunnel: [w366 w373] -> w348
                    frame 0, Default {
                      n258 = call "dvp Vi Get Image Data Gray.vi"("handle"=w371, "pbuffer"=w372) -> ("piHeight out"=w370:i32, "function return"=w367:bool, "pformat out"=w368:i32, "pbuffer out"=w369:u8[], "piWidth out"=w366:i32)  [unwired: 9 in]
                    }
                    frame 1 {
                      n259 = call "dvp Vi Get Image Data Rgb.vi"("handle"=w378, "pbuffer"=w379) -> ("piHeight out"=w374:i32, "function return"=w377:bool, "pformat out"=w375:i32, "pbuffer out"=w376:u32[], "piWidth out"=w373:i32)  [unwired: 9 in]
                    }
                  }
                  n260 = event shown="[2] \"Set 3\": 鼠标按下" {
                    selector: _ -> [_ _ _]
                    dyn-events: _ -> [_ _ _]
                    timeout: 1 -> [_ _ _]
                    tunnel: w355 -> [w412 _ w419]
                    event "Close 3": Mouse Down {
                      n261 = event-data() -> ()  [unwired: 1 in, 5 out]
                      n262 = call "dvp Vi Stop.vi"("handle"=w412) -> ("function return"=w413:u32)  [unwired: 10 in]
                      n263 = case shown="1" w413 {
                        tunnel: w412 -> [_ w416]
                        frame 0, Default {
                        }
                        frame 1 {
                          w415 = T3."Disabled and Grayed Out" ("禁用")
                          n264 = call "dvp Vi Close.vi"("handle"=w416) -> ()  [unwired: 10 in, 1 out]
                          n265 = local write "handle 3"(u32 0 ("handle")) -> ()
                          n266 = property on="Open 3" class="Bool"("DisabledEnum"=T3."Enabled" ("禁用")) -> ()  [unwired: 2 in, 2 out]
                          n267 = local write "CloseFlg 3"(0 ("CloseFlg")) -> ()
                          n268 = property on="Close 3" class="Bool"("DisabledEnum"=w415) -> ()  [unwired: 2 in, 2 out]
                          n269 = property on="Set 3" class="Bool"("DisabledEnum"=w415) -> ()  [unwired: 2 in, 2 out]
                        }
                      }
                    }
                    event Timeout {
                      n270 = event-data() -> ()  [unwired: 1 in, 3 out]
                    }
                    event "Set 3": Mouse Down {
                      n271 = event-data() -> ()  [unwired: 1 in, 8 out]
                      n272 = call "dvp Vi Show Property Modal Dialog.vi"("handle"=w419) -> ()  [unwired: 10 in, 1 out]
                    }
                  }
                  n273 = case shown="真" w352 {
                    tunnel: w348 -> [_ w397]
                    tunnel: w351 -> [_ w396]
                    tunnel: w350 -> [_ w395]
                    tunnel: w349 -> [_ w394]
                    tunnel: w362 -> [_ w393]
                    tunnel: w361 -> [_ w392]
                    tunnel: w360 -> [_ w391]
                    tunnel: w359 -> [_ w390]
                    frame False {
                    }
                    frame True {
                      n274 = case shown="0, 默认" w394 {
                        tunnel: w396 -> [w404 w410]
                        tunnel: w397 -> [w403 w411]
                        tunnel: [w402 w408] -> w389
                        tunnel: w395 -> [w398 w407]
                        tunnel: w393 -> [w400 _]
                        tunnel: w392 -> [w399 _]
                        tunnel: w391 -> [_ w406]
                        tunnel: w390 -> [_ w405]
                        frame 0, Default {
                          n275 = Reshape Array ("重排数组维数")(w398, w404, w403) -> (w401:u32[][])
                          n276 = call "IMAQ ArrayToImage"("error in (no error)"=w399, "Image Pixels (U8)"=w401, "Image"=w400) -> ("Image Out"=w402:T2)  [unwired: 7 in, 1 out]
                        }
                        frame 1 {
                          n277 = Reshape Array ("重排数组维数")(w407, w410, w411) -> (w409:u32[][])
                          n278 = call "IMAQ ArrayToColorImage"("Image Pixels (U32)"=w409, "Image"=w406, "error in (no error)"=w405) -> ("Image Out"=w408:T2)  [unwired: 2 in, 1 out]
                        }
                      }
                      "Image 3" <- w389
                      n279 = local read "Millisecond timing value 6"() -> (w386:u32)
                      n280 = local read "value 4"() -> (w383:u64)
                      n281 = Tick Count (ms)() -> (millisecond timer value=w385:u32)
                      n282 = local read "value 4"() -> (w387:u64)
                      n283 = Increment(x=w383) -> (x+1=w384:u64)
                      n284 = Subtract(x=w385, y=w386) -> (x-y=w380:u32)
                      n285 = local write "value 4"(w384) -> ()
                      n286 = Multiply(x=w387, y=u64 1000) -> (x*y=w382:u64)
                      n287 = Divide(x=w382, y=w380) -> (x/y=w388:dbl)
                      n288 = local write "frame rate"(w388) -> ()
                    }
                  }
                  n289 = local read "CloseFlg 3"() -> (w363:i32)
                  n290 = Equal To 0?(x=w363) -> (x = 0?=w364:bool)
                  n291 = call "dvp Vi Get Frame Count.vi"("handle"=w355) -> ("pFrameCount out"=→"pFrameCount out 3":T1)  [unwired: 9 in, 1 out]
                  n292 = property on="fFrameRate" class="DigNum (严格)"() -> ("Value"=→"Capture frame rate 3":sgl)  [unwired: 2 in, 2 out]
                  n293 = property on="uFrameCount" class="DigNum (严格)"() -> ("Value"=→"Total frame rate 3":u32)  [unwired: 2 in, 2 out]
                }
                n294 = property on="Set 3" class="Bool"("DisabledEnum"=w347) -> ()  [unwired: 2 in, 2 out]
                n295 = property on="Close 3" class="Bool"("DisabledEnum"=w347) -> ()  [unwired: 2 in, 2 out]
                n296 = property on="Open 3" class="Bool"("DisabledEnum"=T3."Disabled and Grayed Out" ("禁用")) -> ()  [unwired: 2 in, 2 out]
              }
            }
            "value 4" <- u64 0 ("数值 4")
          }
        }
      }
      event Application Instance Close {
        n297 = event-data() -> ()  [unwired: 1 in, 4 out]
        n298 = local read "handle 3"() -> (w420:u32)
        n299 = Greater Than 0?(x=w420) -> (x > 0?=w421:bool)
        n300 = case shown="真" w421 {
          tunnel: w420 -> [_ w424]
          frame False {
          }
          frame True {
            n301 = call "dvp Vi Close.vi"("handle"=w424) -> ()  [unwired: 10 in, 1 out]
            n302 = local write "handle 3"(u32 0 ("handle")) -> ()
          }
        }
        n303 = One Button Dialog(message="Exit" ("消息")) -> ()  [unwired: 1 in, 1 out]
      }
    }
  }
  n304 = while {
    stop <- FALSE stop-if-true
    n305 = event shown="[2] \"Open 4\": 鼠标按下" {
      selector: _ -> [_ _ _ _]
      dyn-events: _ -> [_ _ _ _]
      timeout: 10 -> [_ _ _ _]
      event Timeout {
        n306 = event-data() -> ()  [unwired: 1 in, 3 out]
      }
      event "ScanCamera 4": Mouse Down {
        n307 = event-data() -> ()  [unwired: 1 in, 8 out]
        n308 = stacked-sequence "清除下拉列表的数据" {
          frame #0 {
            n309 = property on="CameraList 4" class="Ring (严格)"() -> ("NumItems"=w427:u32)  [unwired: 2 in, 2 out]
            n310 = for {
              N: w427 -> [_]
              n311 = property on="CameraList 4" class="Ring (严格)"() -> ("Value"=w429:u16)  [unwired: 2 in, 2 out]
              n312 = property on="CameraList 4" class="Ring (严格)"() -> ("Strings []"=w428:string[])  [unwired: 2 in, 2 out]
              n313 = Delete From Array ("删除数组元素")(array=w428, index=w429) -> (array with subset deleted=w430:string[])  [unwired: 1 in, 1 out]
              n314 = property on="CameraList 4" class="Ring (严格)"("Strings []"=w430) -> ()  [unwired: 2 in, 2 out]
            }
          }
          frame #1 {
            n315 = call "dvp Vi Refresh.vi"() -> ("pCount out"=w432:u32)  [unwired: 10 in, 1 out]
            n316 = Greater Than 0?(x=w432) -> (x > 0?=w431:bool)
            n317 = case shown="真" w431 {
              tunnel: w432 -> [_ w433]
              frame False {
              }
              frame True {
                n318 = stacked-sequence {
                  tunnel: w433 -> [_ w440]
                  frame #0 {
                    w434 = u32 0 ("index")
                    n319 = property on="CameraList 4" class="Ring (严格)"() -> ("Strings []"=w437:string[])  [unwired: 2 in, 2 out]
                    n320 = call "dvp Vi Enum.vi"("unSize"=u32 64, "index"=w434) -> ("friendlyName out"=w436:string)  [unwired: 8 in, 1 out]
                    n321 = Replace Array Subset ("替换数组子集")(array=w437, new element=w436, index=w434) -> (w438:string[])
                    n322 = property on="CameraList 4" class="Ring (严格)"("Strings []"=w438) -> ()  [unwired: 2 in, 2 out]
                  }
                  frame #1 {
                    n323 = property on="CameraList 4" class="Ring (严格)"() -> ("StringsAndValues[]"=w442:T4)  [unwired: 2 in, 2 out]
                    n324 = Decrement(x=w440) -> (x-1=w439:u32)
                    n325 = for {
                      N: w439 -> [_]
                      shift-right: [w449] -> w441
                      shift-left: w442 -> [w447]
                      i -> [w444]
                      n326 = Increment(x=w444) -> (x+1=w443:i32)
                      n327 = call "dvp Vi Enum.vi"("unSize"=u32 64, "index"=w443) -> ("friendlyName out"=w450:string)  [unwired: 8 in, 1 out]
                      n328 = To Unsigned Word Integer(number=w443) -> (unsigned 16bit integer=w446:u16)
                      n329 = Bundle("friendlyName out"=w450, w446) -> (w448:cluster{"friendlyName out":string, u16})  [unwired: 1 in]
                      n330 = Build Array (concatenate) ("创建数组")(w447, w448) -> (w449:T4)
                    }
                    n331 = property on="CameraList 4" class="Ring (严格)"("StringsAndValues[]"=w441) -> ()  [unwired: 2 in, 2 out]
                  }
                }
              }
            }
          }
        }
      }
      event "Open 4": Mouse Down {
        w453 = u32 1 items=["OPEN_OFFLINE", "OPEN_NORMAL"] ("type")
        n332 = event-data() -> ()  [unwired: 1 in, 8 out]
        n333 = property on="CameraList 4" class="Ring (严格)"() -> ("RingText.Text"=w452:string)  [unwired: 2 in, 2 out]
        n334 = local write "CloseFlg 4"(0 ("CloseFlg")) -> ()
        n335 = call "dvp Vi Open By Name.vi"("type"=w453, "friendlyName"=w452) -> ("pHandle out"=w455:u32, "function return"=w454:u32)  [unwired: 7 in, 1 out]
        n336 = case shown="1" w454 {
          tunnel: w455 -> [_ w458]
          frame 0, Default {
            n337 = One Button Dialog(message="Open Camera fail" ("消息")) -> ()  [unwired: 1 in, 1 out]
          }
          frame 1 {
            n338 = local write "CloseFlg 4"(1 ("CloseFlg")) -> ()
            n339 = local write "handle 4"(w458) -> ()
            n340 = call "dvp Vi Start.vi"("handle"=w458) -> ("function return"=w460:u32)  [unwired: 10 in]
            n341 = call "dvp Vi Set Trigger State.vi"("TriggerState"=0, "handle"=w458) -> ()  [unwired: 9 in, 1 out]
            n342 = case shown="1" w460 {
              tunnel: w458 -> [w465 w479]
              frame 0, Default {
                w464 = T3."Disabled and Grayed Out" ("禁用")
                n343 = local write "handle 4"(u32 0 ("handle")) -> ()
                n344 = local write "CloseFlg 4"(0 ("CloseFlg")) -> ()
                n345 = call "dvp Vi Close.vi"("handle"=w465) -> ()  [unwired: 10 in, 1 out]
                n346 = property on="Set 4" class="Bool"("DisabledEnum"=w464) -> ()  [unwired: 2 in, 2 out]
                n347 = property on="Close 4" class="Bool"("DisabledEnum"=w464) -> ()  [unwired: 2 in, 2 out]
              }
              frame 1 {
                w474 = T5 4 items=["Grayscale (U8)", "Grayscale (I16)", "Grayscale (SGL)", "Complex (CSG)", "RGB (U32)", "HSL (U32)", "RGB (U64)", "Grayscale (U16)"] ("Image Type")
                w477 = T5 0 items=["Grayscale (U8)", "Grayscale (I16)", "Grayscale (SGL)", "Complex (CSG)", "RGB (U32)", "HSL (U32)", "RGB (U64)", "Grayscale (U16)"] ("Image Type")
                w483 = T3."Enabled" ("禁用")
                n348 = Tick Count (ms)() -> (millisecond timer value=→"Millisecond timing value 7":u32)
                n349 = call "dvp Vi Get Image Size.vi"("handle"=w479) -> ("pformat out"=w466:i32, "function return"=w478:u32)  [unwired: 9 in]
                n350 = call "IMAQ Create"("Border Size"=3, "Image Name"="untitled", "Image Type"=w474) -> ("New Image"=w471:T2, "error out"=w470:errorcluster)  [unwired: 2 in]
                n351 = call "IMAQ Create"("Border Size"=3, "Image Name"="untitled4", "Image Type"=w477) -> ("New Image"=w469:T2, "error out"=w468:errorcluster)  [unwired: 2 in]
                n352 = Initialize Array(u8 0 ("元素"), w478) -> (w480:u8[])
                n353 = while {
                  shift-right: [w489] -> _
                  shift-left: w479 -> [w489]
                  tunnel: w480 -> [w491]
                  tunnel: w471 -> [w498]
                  tunnel: w470 -> [w497]
                  tunnel: w469 -> [w496]
                  tunnel: w468 -> [w495]
                  tunnel: w466 -> [w490]
                  stop <- w500 stop-if-true
                  n354 = case shown="0, 默认" w490 {
                    tunnel: w491 -> [w508 w515]
                    tunnel: w489 -> [w507 w514]
                    tunnel: [w503 w513] -> w488
                    tunnel: [w505 w512] -> w487
                    tunnel: [w504 w511] -> w486
                    tunnel: [w506 w510] -> w485
                    tunnel: [w502 w509] -> w484
                    frame 0, Default {
                      n355 = call "dvp Vi Get Image Data Gray.vi"("handle"=w507, "pbuffer"=w508) -> ("piHeight out"=w506:i32, "function return"=w503:bool, "pformat out"=w504:i32, "pbuffer out"=w505:u8[], "piWidth out"=w502:i32)  [unwired: 9 in]
                    }
                    frame 1 {
                      n356 = call "dvp Vi Get Image Data Rgb.vi"("handle"=w514, "pbuffer"=w515) -> ("piHeight out"=w510:i32, "function return"=w513:bool, "pformat out"=w511:i32, "pbuffer out"=w512:u32[], "piWidth out"=w509:i32)  [unwired: 9 in]
                    }
                  }
                  n357 = event shown="[2] \"Set 4\": 鼠标按下" {
                    selector: _ -> [_ _ _]
                    dyn-events: _ -> [_ _ _]
                    timeout: 1 -> [_ _ _]
                    tunnel: w489 -> [w548 _ w555]
                    event "Close 4": Mouse Down {
                      n358 = event-data() -> ()  [unwired: 1 in, 5 out]
                      n359 = call "dvp Vi Stop.vi"("handle"=w548) -> ("function return"=w549:u32)  [unwired: 10 in]
                      n360 = case shown="1" w549 {
                        tunnel: w548 -> [_ w552]
                        frame 0, Default {
                        }
                        frame 1 {
                          w551 = T3."Disabled and Grayed Out" ("禁用")
                          n361 = call "dvp Vi Close.vi"("handle"=w552) -> ()  [unwired: 10 in, 1 out]
                          n362 = local write "handle 4"(u32 0 ("handle")) -> ()
                          n363 = property on="Open 4" class="Bool"("DisabledEnum"=T3."Enabled" ("禁用")) -> ()  [unwired: 2 in, 2 out]
                          n364 = local write "CloseFlg 4"(0 ("CloseFlg")) -> ()
                          n365 = property on="Close 4" class="Bool"("DisabledEnum"=w551) -> ()  [unwired: 2 in, 2 out]
                          n366 = property on="Set 4" class="Bool"("DisabledEnum"=w551) -> ()  [unwired: 2 in, 2 out]
                        }
                      }
                    }
                    event Timeout {
                      n367 = event-data() -> ()  [unwired: 1 in, 3 out]
                    }
                    event "Set 4": Mouse Down {
                      n368 = event-data() -> ()  [unwired: 1 in, 8 out]
                      n369 = call "dvp Vi Show Property Modal Dialog.vi"("handle"=w555) -> ()  [unwired: 10 in, 1 out]
                    }
                  }
                  n370 = case shown="真" w488 {
                    tunnel: w484 -> [_ w533]
                    tunnel: w485 -> [_ w532]
                    tunnel: w487 -> [_ w530]
                    tunnel: w486 -> [_ w529]
                    tunnel: w498 -> [_ w528]
                    tunnel: w497 -> [_ w527]
                    tunnel: w496 -> [_ w526]
                    tunnel: w495 -> [_ w525]
                    frame False {
                    }
                    frame True {
                      n371 = case shown="0, 默认" w529 {
                        tunnel: w532 -> [w540 w546]
                        tunnel: w533 -> [w539 w547]
                        tunnel: [w538 w544] -> w531
                        tunnel: w530 -> [w534 w543]
                        tunnel: w528 -> [_ w542]
                        tunnel: w527 -> [_ w541]
                        tunnel: w526 -> [w536 _]
                        tunnel: w525 -> [w535 _]
                        frame 0, Default {
                          n372 = Reshape Array ("重排数组维数")(w534, w540, w539) -> (w537:u32[][])
                          n373 = call "IMAQ ArrayToImage"("error in (no error)"=w535, "Image Pixels (U8)"=w537, "Image"=w536) -> ("Image Out"=w538:T2)  [unwired: 7 in, 1 out]
                        }
                        frame 1 {
                          n374 = Reshape Array ("重排数组维数")(w543, w546, w547) -> (w545:u32[][])
                          n375 = call "IMAQ ArrayToColorImage"("Image Pixels (U32)"=w545, "Image"=w542, "error in (no error)"=w541) -> ("Image Out"=w544:T2)  [unwired: 2 in, 1 out]
                        }
                      }
                      "Image 4" <- w531
                      n376 = local read "Millisecond timing value 7"() -> (w518:u32)
                      n377 = local read "value 5"() -> (w521:u64)
                      n378 = Tick Count (ms)() -> (millisecond timer value=w519:u32)
                      n379 = local read "value 5"() -> (w517:u64)
                      n380 = Increment(x=w521) -> (x+1=w520:u64)
                      n381 = Subtract(x=w519, y=w518) -> (x-y=w524:u32)
                      n382 = local write "value 5"(w520) -> ()
                      n383 = Multiply(x=w517, y=u64 1000) -> (x*y=w522:u64)
                      n384 = Divide(x=w522, y=w524) -> (x/y=w516:dbl)
                      n385 = local write "frame rate"(w516) -> ()
                    }
                  }
                  n386 = local read "CloseFlg 4"() -> (w499:i32)
                  n387 = Equal To 0?(x=w499) -> (x = 0?=w500:bool)
                  n388 = call "dvp Vi Get Frame Count.vi"("handle"=w489) -> ("pFrameCount out"=→"pFrameCount out 4":T1)  [unwired: 9 in, 1 out]
                  n389 = property on="fFrameRate" class="DigNum (严格)"() -> ("Value"=→"Capture frame rate 4":sgl)  [unwired: 2 in, 2 out]
                  n390 = property on="uFrameCount" class="DigNum (严格)"() -> ("Value"=→"Total frame rate 4":u32)  [unwired: 2 in, 2 out]
                }
                n391 = property on="Set 4" class="Bool"("DisabledEnum"=w483) -> ()  [unwired: 2 in, 2 out]
                n392 = property on="Close 4" class="Bool"("DisabledEnum"=w483) -> ()  [unwired: 2 in, 2 out]
                n393 = property on="Open 4" class="Bool"("DisabledEnum"=T3."Disabled and Grayed Out" ("禁用")) -> ()  [unwired: 2 in, 2 out]
              }
            }
            "value 5" <- u64 0 ("数值 5")
          }
        }
      }
      event Application Instance Close {
        n394 = event-data() -> ()  [unwired: 1 in, 4 out]
        n395 = local read "handle 4"() -> (w556:u32)
        n396 = Greater Than 0?(x=w556) -> (x > 0?=w557:bool)
        n397 = case shown="真" w557 {
          tunnel: w556 -> [_ w560]
          frame False {
          }
          frame True {
            n398 = call "dvp Vi Close.vi"("handle"=w560) -> ()  [unwired: 10 in, 1 out]
            n399 = local write "handle 4"(u32 0 ("handle")) -> ()
          }
        }
        n400 = One Button Dialog(message="Exit" ("消息")) -> ()  [unwired: 1 in, 1 out]
      }
    }
  }
  "handle" <- u32 0 ("handle")
  "handle 2" <- u32 0 ("handle")
  "handle 3" <- u32 0 ("handle")
  "handle 4" <- u32 0 ("handle")
  "frame rate" <- 0.0 ("帧率")
  "frame rate" <- 0.0 ("帧率 3")
  "frame rate" <- 0.0 ("帧率 4")
  "frame rate" <- 0.0 ("帧率 2")
